vi "KepcoDCPwr Configure List Angle.vi"(0 "VISA Session":refnum<visa-resource-name>, 2 "List Type (DWell)":enum16{"Current List", "Voltage List"}(ring)=enum."Voltage List", 5 "Model In":string, 7 "channel name (\"\")":string="\"\"", 11 "error in (no error)":errorcluster {"code" format="%.0x"}, 12 "Start degree":dbl=1.0 min=0.0 max=255.0, 13 "End degree":dbl=1.0 min=0.0 max=255.0) -> (4 "VISA Session Out":refnum<visa-resource-name>, 6 "Model Out":string, 8 "channel name out (\"\")":string="\"\"" caption="channel name Out (\"\")", 15 "error out":errorcluster {"code" format="%.0x"})   [LabVIEW 2013]
doc: "This VI Sets List start and end angle for a Sine or Triangle Waveform segment. \n\n\nNotE:\n1) This VI does not change operational status of Power supply\n2. This Vi should be used before sending the segment.\n3.) Start and End angle is a value from 0 to 360 degrees. The difference between the Start and end angle must be no greater than 360 degrees.\n4. Clear All List (List CLEAR command) sets start and end to 0 and 360."
uses:
  <vilib>/regexp/Match Regular Expression.xnode
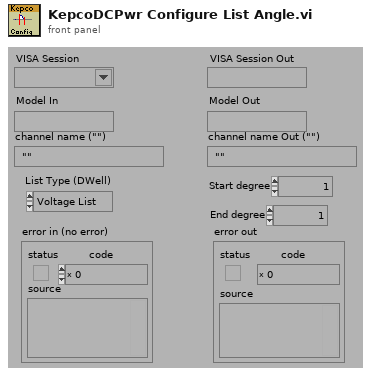
[diagram p1: front panel]
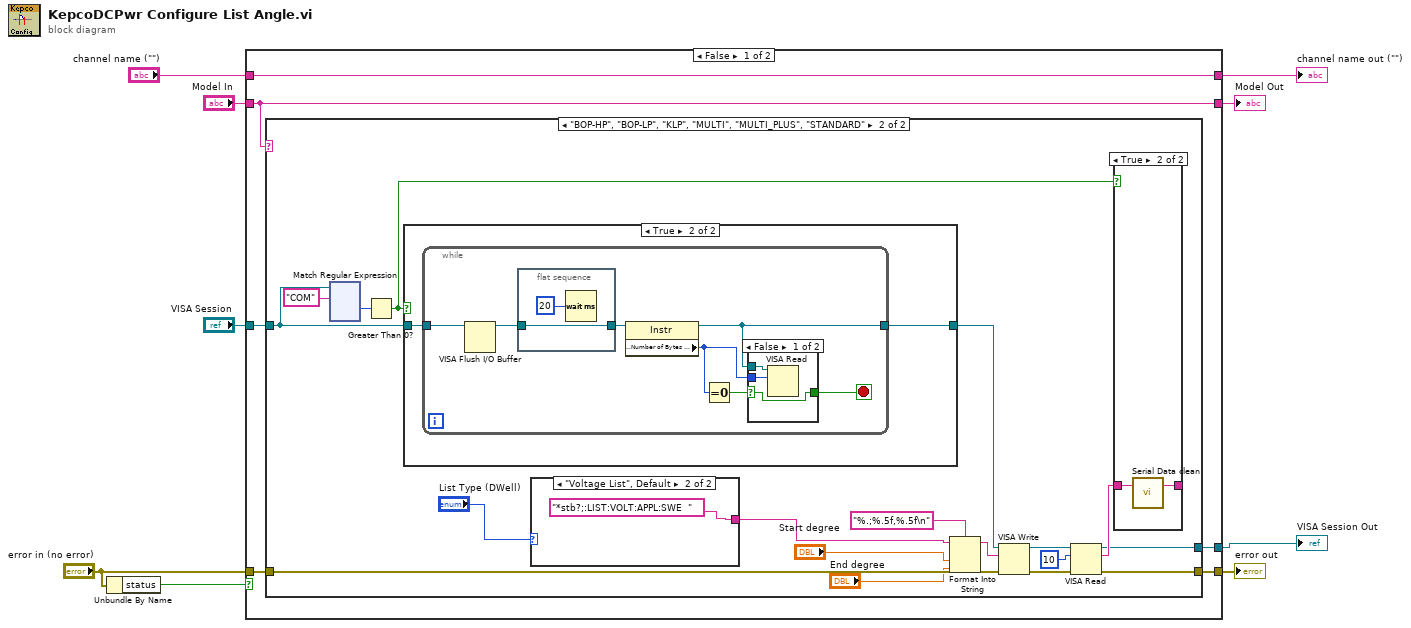
[diagram p0: block diagram]
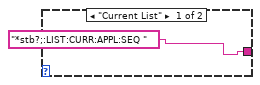
[diagram p3: hidden frame]
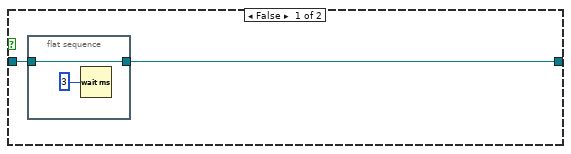
[diagram p5: hidden frame]
diagram:
  n1 = Unbundle By Name("error in (no error)") -> ("status"=w8:bool)
  n2 = case shown="False" w8 {
    tunnel: [w11 w174] -> w9
    tunnel: "error in (no error)" -> [w10 w174]
    tunnel: [w12 w173] -> w1
    tunnel: "VISA Session" -> [w13 w173]
    tunnel: [w14 w172] -> w2
    tunnel: "Model In" -> [w14 w172]
    tunnel: [w15 w171] -> w3
    tunnel: "channel name (\"\")" -> [w15 w171]
    frame False {
      n3 = case shown="\"BOP-HP\", \"BOP-LP\", \"KLP\", \"MULTI\", \"MULTI_PLUS\", \"STANDARD\"" w14 {
        tunnel: w10 -> [w17 w29]
        tunnel: [w17 w23] -> w11
        tunnel: w13 -> [w16 w33]
        tunnel: [w16 w24] -> w12
        frame "", Default {
        }
        frame "BOP-HP", "BOP-LP", "KLP", "MULTI", "MULTI_PLUS", "STANDARD" {
          n4 = xnode "Match Regular Expression"("input string"=w33, "regular expression"="COM") -> ("offset past match"=w34:i32)  [unwired: 2 in, 6 out]
          n5 = Greater Than 0?(x=w34) -> (x > 0?=w32:bool)
          n6 = case shown="True" w32 {
            tunnel: [w42 w46] -> w30
            tunnel: w33 -> [w41 w45]
            frame False {
              n7 = flat-sequence {
                tunnel: w41 -> [w44]
                tunnel: [w44] -> w42
                frame #0 {
                  n8 = Wait (ms)(milliseconds to wait=u32 3 ("byte count (0)")) -> ()  [unwired: 1 out]
                }
              }
            }
            frame True {
              n9 = while {
                tunnel: w45 -> [w49]
                tunnel: [w51] -> w46
                stop <- w52 stop-if-true
                n10 = VISA Flush I/O Buffer(VISA resource name=w49) -> (VISA resource name out=w48:refnum<visa-resource-name>)  [unwired: 2 in, 1 out]
                n11 = flat-sequence {
                  tunnel: w48 -> [w54]
                  tunnel: [w54] -> w47
                  frame #0 {
                    n12 = Wait (ms)(milliseconds to wait=u32 20) -> ()  [unwired: 1 out]
                  }
                }
                n13 = property class="Instr"(reference=w47) -> (reference out=w51:refnum<visa-resource-name>, "Serial Settings:Number of Bytes at Serial Port"=w50:u32)  [unwired: 1 in, 1 out]
                n14 = Equal To 0?(x=w50) -> (x = 0?=w53:bool)
                n15 = case shown="False" w53 {
                  selector: w53 -> [w58 w59]
                  tunnel: [w58 w59] -> w52
                  tunnel: w51 -> [w57 _]
                  tunnel: w50 -> [w56 _]
                  frame False {
                    n16 = VISA Read(VISA resource name=w57, byte count=w56) -> ()  [unwired: 1 in, 4 out]
                  }
                  frame True {
                  }
                }
              }
            }
          }
          n17 = case shown="\"Voltage List\", Default" "List Type (DWell)" {
            tunnel: ["*stb?;:LIST:CURR:APPL:SEQ " "*stb?;:LIST:VOLT:APPL:SWE  "] -> w21
            frame "Current List" {
            }
            frame "Voltage List", Default {
            }
          }
          n18 = Format Into String(format string="%.;%.5f,%.5f\n", initial string=w21, "Start degree", "End degree") -> (resulting string=w31:string)  [unwired: 1 in, 1 out]
          n19 = VISA Write(VISA resource name=w30, write buffer=w31, error in (no error)=w29) -> (VISA resource name out=w28:refnum<visa-resource-name>, error out=w27:errorcluster)  [unwired: 1 out]
          n20 = VISA Read(VISA resource name=w28, byte count=u32 10, error in (no error)=w27) -> (VISA resource name out=w24:refnum<visa-resource-name>, read buffer=w25:string, error out=w23:errorcluster)  [unwired: 1 out]
          n21 = case shown="True" w32 {
            tunnel: w25 -> [w38 w39]
            tunnel: [w38 w40] -> _
            frame False {
            }
            frame True {
              n22 = call "Serial Data clean.vi"("string"=w39) -> ("Stripped of Xon Xoff"=w40:string)  [unwired: 2 in]
            }
          }
        }
      }
    }
    frame True {
    }
  }
  "error out" <- w9
  "channel name out (\"\")" <- w3
  "Model Out" <- w2
  "VISA Session Out" <- w1
